vi "Tbl Comp.vi"(5 "배열":refnum<vi>[](array[refnum]), 7 "방향":enum16{"수직", "수평"}(ring), 8 "에러 입력":errorcluster caption="에러 입력(에러 없음)") -> (0 "에러 출력":errorcluster, 1 "Right":i32, 2 "Top":i32)   [LabVIEW 2020]
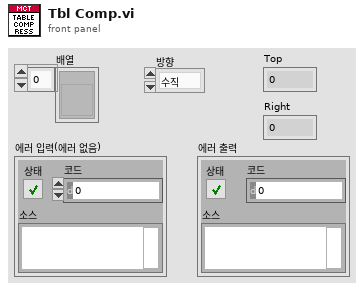
[diagram p1: front panel]
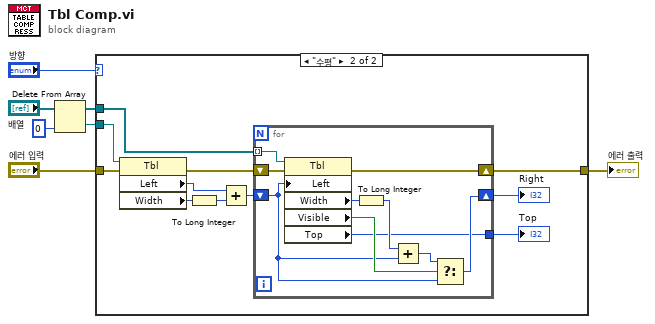
[diagram p0: block diagram]
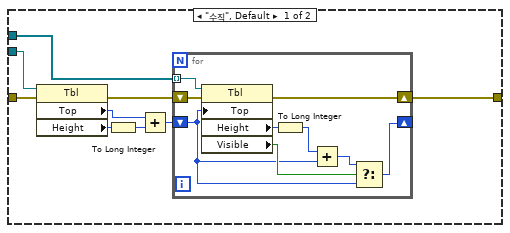
[diagram p2: hidden frame]
diagram:
  n1 = Delete From Array(array="배열", index=0 ("인덱스")) -> (deleted portion=w2:refnum<vi>, array with subset deleted=w4:refnum<vi>[])  [unwired: 1 in]
  n2 = case shown="\"수평\"" "방향" {
    tunnel: [w10 w36] -> w7
    tunnel: "에러 입력" -> [w11 w35]
    tunnel: w4 -> [w9 w33]
    tunnel: w2 -> [w8 w32]
    frame "수직", Default {
      n3 = property class="Tbl"(reference=w8, error in=w11) -> (error out=w12:errorcluster, "Top"=w13:i32, "Height"=w14:u32)  [unwired: 1 out]
      n4 = To Long Integer(number=w14) -> (32bit integer=w16:i32)
      n5 = Add(x=w13, y=w16) -> (x+y=w15:i32)
      n6 = for {
        tunnel: w9 -> [w24] mode=indexing
        shift-right: [w23] -> w10
        shift-left: w12 -> [w25]
        shift-right: [w17] -> _
        shift-left: w15 -> [w18]
        n7 = property class="Tbl"(reference=w24, error in=w25, "Top"=w18) -> (error out=w23:errorcluster, "Height"=w22:u32, "Visible"=w20:bool)  [unwired: 1 out]
        n8 = To Long Integer(number=w22) -> (32bit integer=w21:i32)
        n9 = Add(x=w21, y=w18) -> (x+y=w19:i32)
        n10 = Select(t=w19, s=w20, f=w18) -> (s? t:f=w17:i32)
      }
    }
    frame "수평" {
      n11 = property class="Tbl"(reference=w32, error in=w35) -> (error out=w34:errorcluster, "Left"=w31:i32, "Width"=w30:u32)  [unwired: 1 out]
      n12 = To Long Integer(number=w30) -> (32bit integer=w28:i32)
      n13 = Add(x=w31, y=w28) -> (x+y=w29:i32)
      n14 = for {
        tunnel: w33 -> [w45] mode=indexing
        shift-right: [w44] -> w36
        shift-left: w34 -> [w46]
        shift-right: [w38] -> w26
        shift-left: w29 -> [w39]
        tunnel: [w37] -> w27
        n15 = property class="Tbl"(reference=w45, error in=w46, "Left"=w39) -> (error out=w44:errorcluster, "Width"=w43:u32, "Visible"=w41:bool, "Top"=w37:i32)  [unwired: 1 out]
        n16 = To Long Integer(number=w43) -> (32bit integer=w42:i32)
        n17 = Add(x=w42, y=w39) -> (x+y=w40:i32)
        n18 = Select(t=w40, s=w41, f=w39) -> (s? t:f=w38:i32)
      }
      "Top" <- w27
      "Right" <- w26
    }
  }
  "에러 출력" <- w7
